vi "Test Stack Operations.vi"() -> ()   [LabVIEW 2013]
uses:
  VariantBuffer/buffer-type -- enum.ctl
  VariantBuffer/VariantBuffer.lvclass
panel:
  out "error out 2":errorcluster
  out "Stack flushed (reverse order)":bool
  out "Stack pushed (array)":bool
  out "Stack full":bool
  out "Stack poppped (reverse order)":bool
  out "error out":errorcluster
  out "Stack pushed":bool
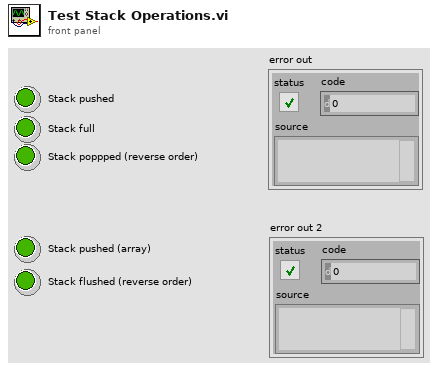
[diagram p1: front panel]
types:
  T1 = typedef "CircularBuffer.lvlib/VariantBuffer.lvclass/buffer-type -- enum.ctl" = enum16{"Queue", "Stack"}
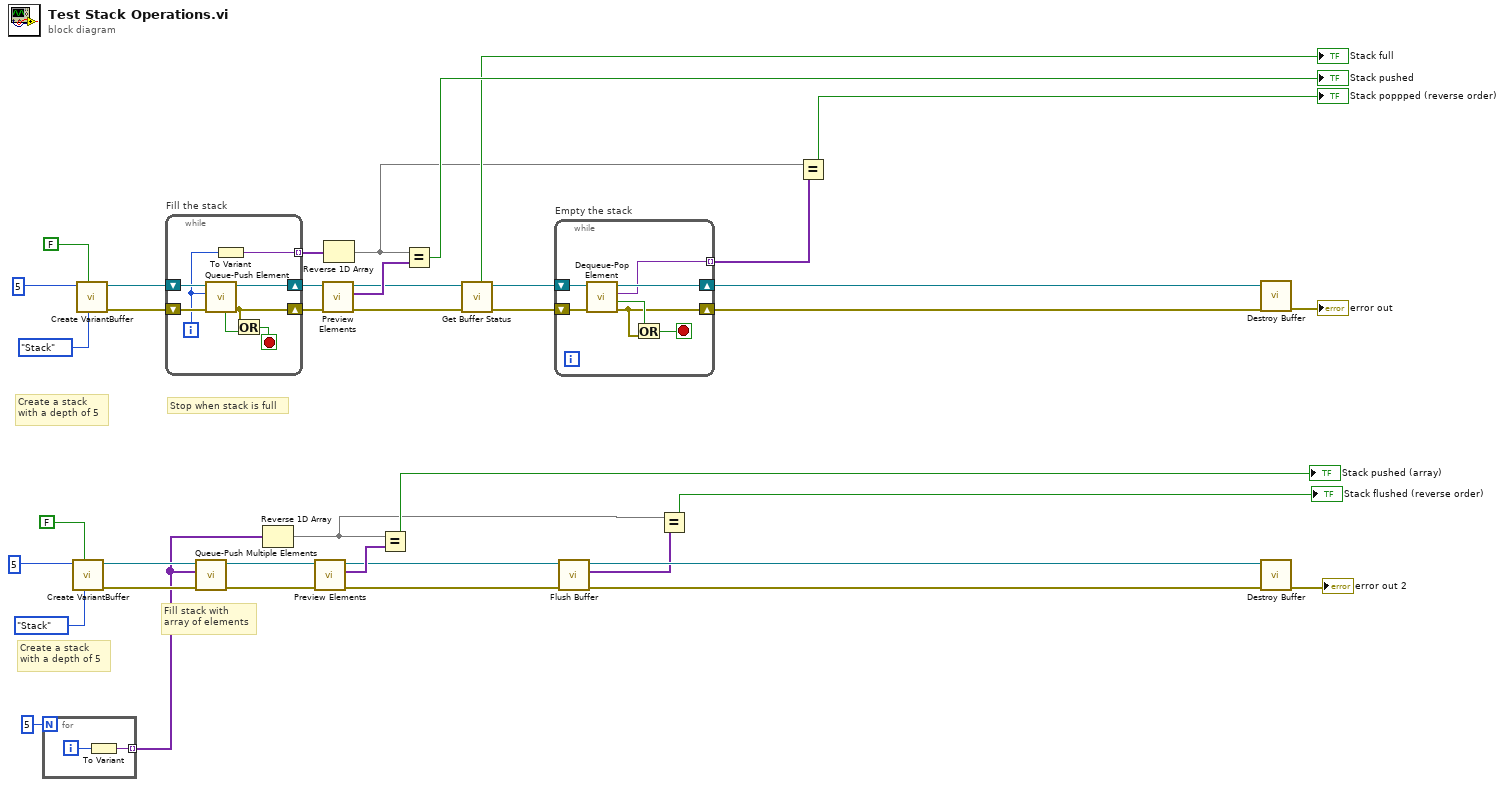
[diagram p0: block diagram]
diagram:
  # "Fill stack with\narray of elements"
  # "Create a stack\nwith a depth of 5"
  # "Stop when stack is full"
  # "Create a stack\nwith a depth of 5"
  n1 = for {
    N: 5 -> [_]
    tunnel: [w41] -> w2 mode=indexing
    i -> [w42]
    n2 = To Variant(anything=w42) -> (Variant=w41:variant)
  }
  n3 = call "Create VariantBuffer.vi"("buffer-type"=buffer-type_--_enum."Stack", "Allow Overflow? (T)"=FALSE, "bufSize"=5) -> ("error out"=w17:errorcluster, "Buffer"=w18:refnum<data-value>)  [unwired: 7 in]
  n4 = call "Create VariantBuffer.vi"("buffer-type"=buffer-type_--_enum."Stack", "Allow Overflow? (T)"=FALSE, "bufSize"=5) -> ("error out"=w37:errorcluster, "Buffer"=w36:refnum<data-value>)  [unwired: 7 in]
  n5 = while "Fill the stack" {
    shift-right: [w43] -> w32
    shift-left: w37 -> [w50]
    shift-right: [w48] -> w34
    shift-left: w36 -> [w49]
    tunnel: [w46] -> w4 mode=indexing
    i -> [w47]
    stop <- w44 stop-if-true
    n6 = call "Queue-Push Element.vi"("error in"=w50, "element"=w47, "Buffer in"=w49) -> ("error out"=w43:errorcluster, "Buffer"=w48:refnum<data-value>, "full"=w45:bool)  [unwired: 4 in, 2 out]
    n7 = To Variant(anything=w47) -> (Variant=w46:variant)
    n8 = Or(x=w43, y=w45) -> (x .or. y?=w44:bool)
  }
  n9 = call "Queue-Push Multiple Elements.vi"("error in"=w17, "elements"=w2, "Buffer in"=w18) -> ("error out"=w14:errorcluster, "Buffer"=w15:refnum<data-value>)  [unwired: 6 in, 1 out]
  n10 = Reverse 1D Array(array=w2) -> (reversed array=w1:variant[])
  n11 = call "Preview Elements.vi"("error in"=w14, "ByteBuffer in"=w15) -> ("error out"=w11:errorcluster, "elements"=w13:variant[], "ByteBuffer"=w12:refnum<data-value>)  [unwired: 7 in]
  n12 = call "Preview Elements.vi"("error in"=w32, "ByteBuffer in"=w34) -> ("error out"=w24:errorcluster, "elements"=w33:variant[], "ByteBuffer"=w26:refnum<data-value>)  [unwired: 7 in]
  n13 = Reverse 1D Array(array=w4) -> (reversed array=w3:variant[])
  n14 = Equal?(x=w1, y=w13) -> (x = y?=→"Stack pushed (array)":bool)
  n15 = Equal?(x=w3, y=w33) -> (x = y?=→"Stack pushed":bool)
  n16 = call "Get Buffer Status.vi"("error in"=w24, "Buffer in"=w26) -> ("error out"=w23:errorcluster, "Buffer"=w25:refnum<data-value>, "full"=→"Stack full":bool)  [unwired: 5 in, 2 out]
  n17 = while "Empty the stack" {
    shift-right: [w55] -> w30
    shift-left: w25 -> [w57]
    shift-right: [w53] -> w29
    shift-left: w23 -> [w56]
    tunnel: [w51] -> w28 mode=indexing
    stop <- w52 stop-if-true
    n18 = call "Dequeue-Pop Element.vi"("error in"=w56, "Buffer in"=w57) -> ("error out"=w53:errorcluster, "buffer empty?"=w54:bool, "element"=w51:variant, "Buffer"=w55:refnum<data-value>)  [unwired: 6 in]
    n19 = Or(x=w54, y=w53) -> (x .or. y?=w52:bool)
  }
  n20 = call "Flush Buffer.vi"("error in"=w11, "Buffer in"=w12) -> ("error out"=w9:errorcluster, "elements"=w8:variant[], "Buffer"=w10:refnum<data-value>)  [unwired: 7 in]
  n21 = Equal?(x=w1, y=w8) -> (x = y?=→"Stack flushed (reverse order)":bool)
  n22 = Equal?(x=w3, y=w28) -> (x = y?=→"Stack poppped (reverse order)":bool)
  n23 = call "Destroy Buffer.vi"("error in"=w29, "Buffer"=w30) -> ("error out"=→"error out":errorcluster)  [unwired: 8 in, 1 out]
  n24 = call "Destroy Buffer.vi"("error in"=w9, "Buffer"=w10) -> ("error out"=→"error out 2":errorcluster)  [unwired: 8 in, 1 out]
